vi "move_4b.vi"(6 "Array 5":i32[](array[numeric]), 7 "Array in":i32[](array[numeric]), 9 "Array 3":i32[](array[numeric]), 10 "Enum 4":T1(ring), 11 "Enum in":enum16{"move4", "move4_1", "move4_2"}(ring)) -> (1 "Array 4":i32[](array[numeric]), 2 "Enum 3":T2(ring), 3 "Enum out":enum16{"move4", "move4_1", "move4_2"}(ring), 4 "Array 6":i32[](array[numeric]), 5 "Array out":i32[](array[numeric]))   [LabVIEW 2016]
uses:
  <vilib>/NXT/Block Support/NXT_OutputPort.ctl
  <vilib>/NXT/NXTIO Xnodes/NXTIONodeSubVIs/NXTStopMotors.vi
  <vilib>/NXT/NXTIO Xnodes/NXTIONodeSubVIs/NXTMotorRunDistance.vi
  <vilib>/NXT/NXTIO Xnodes/NXTIONodeSubVIs/LEGOMotorStatus.vi
  <vilib>/NXT/NXTIO Xnodes/NXTIONodeSubVIs/NXTMoveMotors.vi
  <vilib>/NXT/NXTIO Xnodes/NXTIONodeSubVIs/LEGOResetMotors.vi
  <vilib>/NXT/Subs/LVHSConnector.ctl
  <vilib>/NXT/NXTIO Xnodes/AddressXNode/NXTIOAddress.xnode
  <vilib>/NXT/NXTIO Xnodes/NXTIOXNode/NXTIO.xnode
  <vilib>/NXT/LegoClasses/BrickReference/BrickReference.lvclass
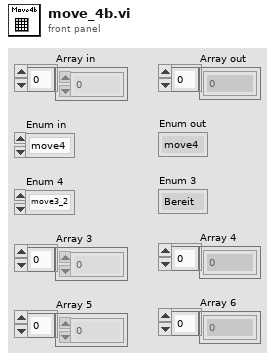
[diagram p1: front panel]
types:
  T1 = enum16{"move3_2", "move3_3", "move3_4", "move3_5"}
  T2 = enum16{"Bereit", "Move 1", "Reference_pos", "Wait", "row1_check", "row2_check", "row3_check", "return", "move2", "move3", "move4", "move5", "end"}
  T3 = enum16{"forward", "right", "mark", "pause", "up", "return", "end"}
  T4 = typedef "NXT_OutputPort.ctl" = u8
  T5 = cluster{"Output Port":T4, "Output Port 2":T4, "Output Port 3":T4}
  T6 = enum16{"forward", "mark", "pause", "up", "return", "end"}
  T7 = typedef "LVHSConnector.ctl" = refnum<class "BrickReference.lvclass">
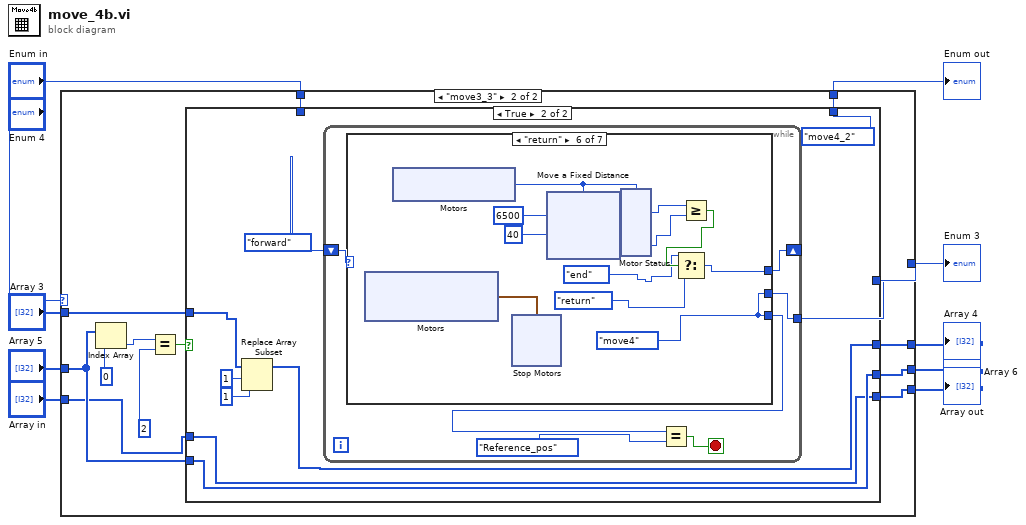
[diagram p0: block diagram]
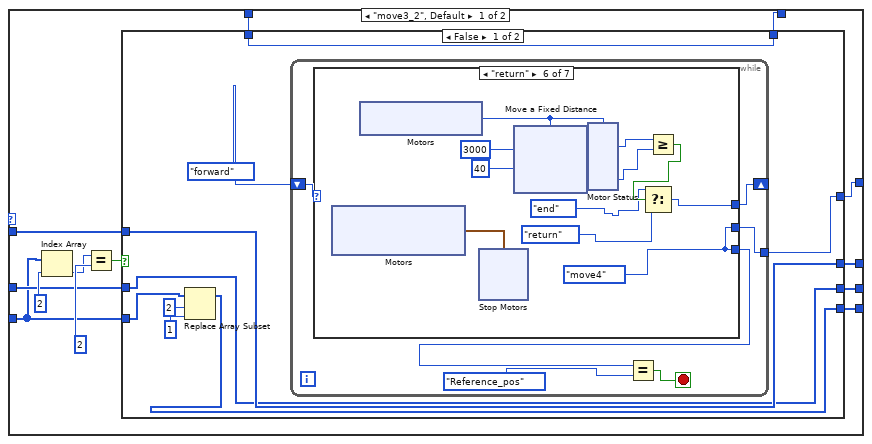
[diagram p2: hidden frame]
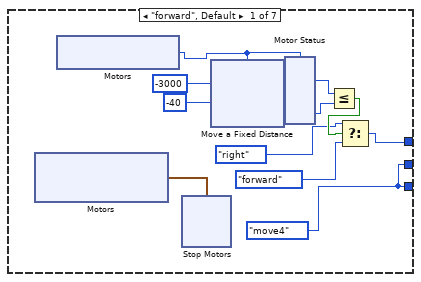
[diagram p3: hidden frame]
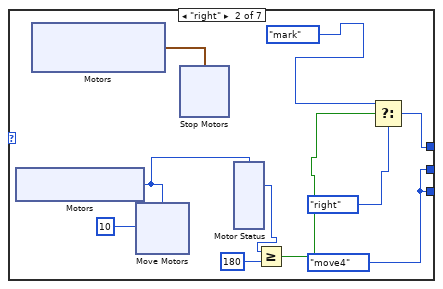
[diagram p4: hidden frame]
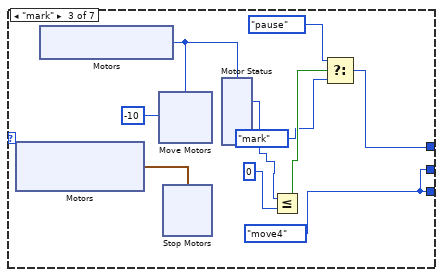
[diagram p5: hidden frame]
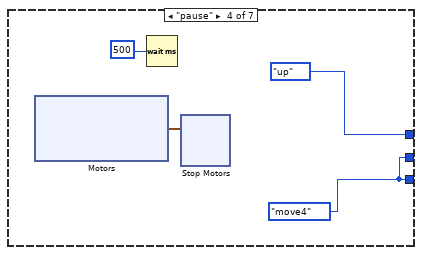
[diagram p6: hidden frame]
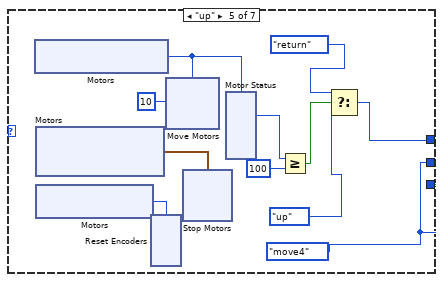
[diagram p7: hidden frame]
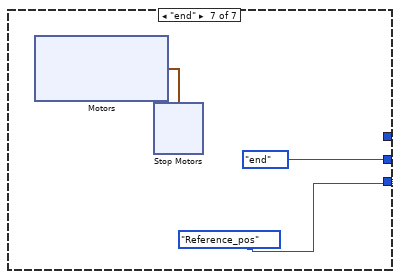
[diagram p8: hidden frame]
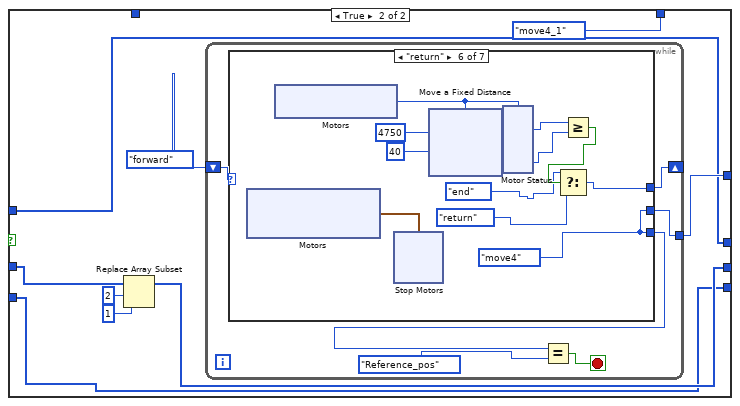
[diagram p9: hidden frame]
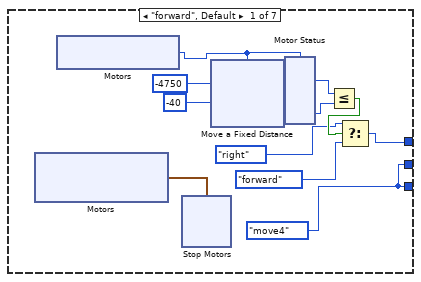
[diagram p10: hidden frame]
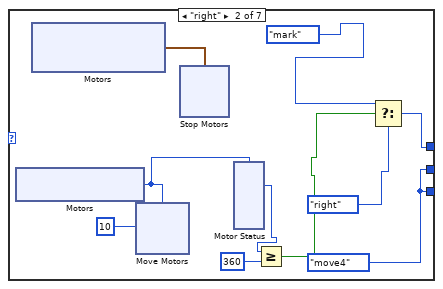
[diagram p11: hidden frame]
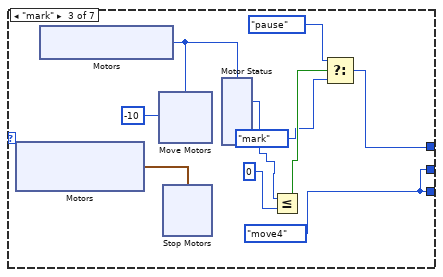
[diagram p12: hidden frame]
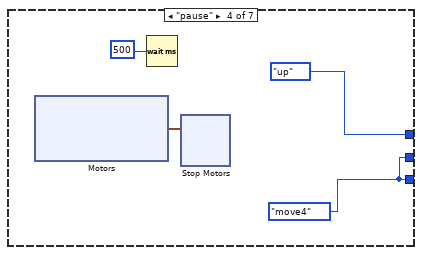
[diagram p13: hidden frame]
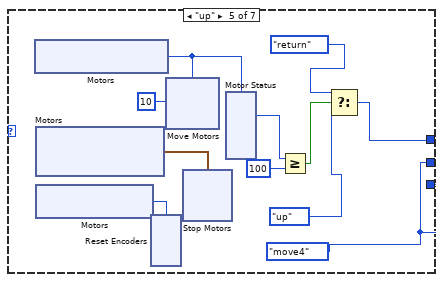
[diagram p14: hidden frame]
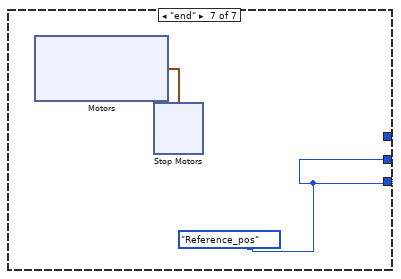
[diagram p15: hidden frame]
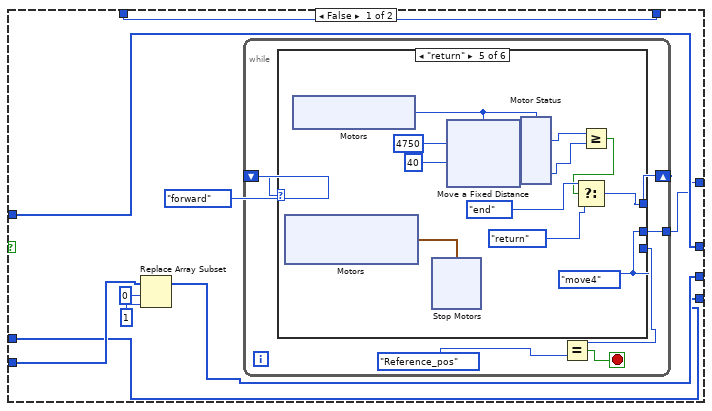
[diagram p16: hidden frame]
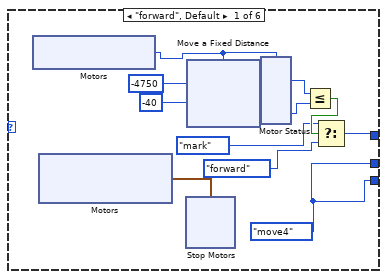
[diagram p17: hidden frame]
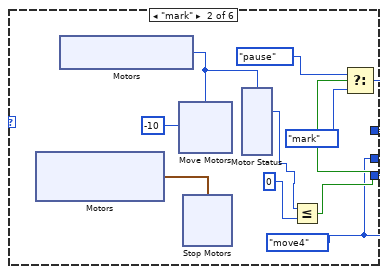
[diagram p18: hidden frame]
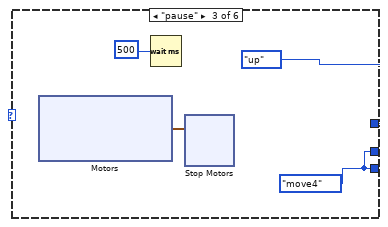
[diagram p19: hidden frame]
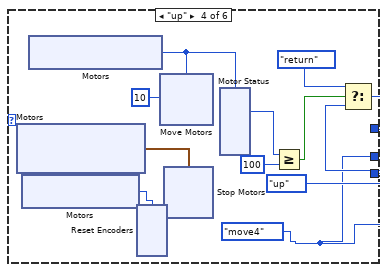
[diagram p20: hidden frame]
diagram:
  n1 = case shown="\"move3_3\"" "Enum 4" {
    tunnel: [w22 w450] -> w2
    tunnel: [w21 w449] -> w3
    tunnel: "Enum in" -> [w20 w448]
    tunnel: [w18 w442] -> w5
    tunnel: "Array 5" -> [w17 w441]
    tunnel: [w14 w443] -> w7
    tunnel: "Array 3" -> [w13 w444]
    tunnel: [w12 w440] -> w9
    tunnel: "Array in" -> [w11 w439]
    frame "move3_2", Default {
      n2 = Index Array(array=w11, index=2) -> (element=w16:i32)
      n3 = Equal?(x=w16, y=2 ("element")) -> (x = y?=w15:bool)
      n4 = case shown="False" w15 {
        tunnel: [w28 w239] -> w22
        tunnel: [w29 enum16{"move4", "move4_1", "move4_2"}."move4_1"] -> w21
        tunnel: w20 -> [w29 _]
        tunnel: [w24 w237] -> w18
        tunnel: w17 -> [w24 w238]
        tunnel: [w27 w233] -> w14
        tunnel: w13 -> [w27 w233]
        tunnel: [w25 w234] -> w12
        tunnel: w11 -> [w26 w234]
        frame False {
          n5 = Replace Array Subset(array=w26, new element=1 ("new element/subarray"), index=2) -> (w25:i32[])
          n6 = while {
            shift-right: [w34] -> _
            shift-left: T3."forward" -> [w35]
            tunnel: [w33] -> w28
            stop <- w37 stop-if-true
            n7 = case shown="\"return\"" w35 {
              tunnel: [w39 w76 w108 T3."up" w151 w187 _] -> w34
              tunnel: [w48 w75 w107 w139 w150 w196 T2."Reference_pos"] -> w38
              tunnel: [w48 w75 w107 w139 w150 w196 T2."end"] -> w33
              frame "forward", Default {
                w44 = -3000 ("Distance 1")
                w48 = T2."move4"
                n8 = xnode "Motors"() -> ("Motor"=w49:cluster{"Port":T4, "Port":T4})
                n9 = xnode "Motors"() -> ("Motor"=w43:T4)
                n10 = xnode "Stop Motors"("Motors"=w49) -> ()  [unwired: 1 in, 1 out]
                n11 = xnode "Move a Fixed Distance"("Speed 1"=i8 -40, "Distance 1"=w44, "Motors"=w43) -> ("NXT/EV3"=w45:T7)  [unwired: 1 in]
                n12 = xnode "Motor Status"("Motors"=w43, "NXT/EV3"=w45) -> ("Position 1"=w46:i32)  [unwired: 2 out]
                n13 = Less Or Equal?(x=w46, y=w44) -> (x <= y?=w42:bool)
                n14 = Select(t=T3."right", s=w42, f=T3."forward") -> (s? t:f=w39:T3)
              }
              frame "right" {
                w75 = T2."move4"
                n15 = xnode "Motors"() -> ("Motor"=w84:T4)
                n16 = xnode "Motors"() -> ("Motor"=w83:cluster{"Port":T4, "Port":T4})
                n17 = xnode "Move Motors"("Power/Speed 1"=i8 10, "Motors"=w84) -> ()  [unwired: 1 in, 1 out]
                n18 = xnode "Stop Motors"("Motors"=w83) -> ()  [unwired: 1 in, 1 out]
                n19 = xnode "Motor Status"("Motors"=w84) -> ("Position 1"=w81:i32)  [unwired: 1 in, 2 out]
                n20 = Greater Or Equal?(x=w81, y=180) -> (x >= y?=w80:bool)
                n21 = Select(t=T3."mark", s=w80, f=T3."right") -> (s? t:f=w76:T3)
              }
              frame "mark" {
                w107 = T2."move4"
                n22 = xnode "Motors"() -> ("Motor"=w116:cluster{"Port":T4, "Port":T4})
                n23 = xnode "Motors"() -> ("Motor"=w114:T4)
                n24 = xnode "Move Motors"("Power/Speed 1"=i8 -10, "Motors"=w114) -> ()  [unwired: 1 in, 1 out]
                n25 = xnode "Stop Motors"("Motors"=w116) -> ()  [unwired: 1 in, 1 out]
                n26 = xnode "Motor Status"("Motors"=w114) -> ("Position 1"=w113:i32)  [unwired: 1 in, 2 out]
                n27 = Less Or Equal?(x=w113, y=0) -> (x <= y?=w111:bool)
                n28 = Select(t=T3."pause", s=w111, f=T3."mark") -> (s? t:f=w108:T3)
              }
              frame "pause" {
                w139 = T2."move4"
                n29 = xnode "Motors"() -> ("Motor"=w142:cluster{"Port":T4, "Port":T4, "Port":T4})
                n30 = Wait (ms)(milliseconds to wait=u32 500 ("millisecond timer value")) -> ()  [unwired: 1 out]
                n31 = xnode "Stop Motors"("Motors"=w142) -> ()  [unwired: 1 in, 1 out]
              }
              frame "up" {
                w150 = T2."move4"
                n32 = xnode "Motors"() -> ("Motor"=w155:T4)
                n33 = xnode "Motors"() -> ("Motor"=w158:cluster{"Port":T4, "Port":T4})
                n34 = xnode "Motors"() -> ("Motor"=w149:T4)
                n35 = xnode "Reset Encoders"("Motors"=w149) -> ()  [unwired: 1 in, 1 out]
                n36 = xnode "Move Motors"("Power/Speed 1"=i8 10, "Motors"=w155) -> ()  [unwired: 1 in, 1 out]
                n37 = xnode "Stop Motors"("Motors"=w158) -> ()  [unwired: 1 in, 1 out]
                n38 = xnode "Motor Status"("Motors"=w155) -> ("Position 1"=w156:i32)  [unwired: 1 in, 2 out]
                n39 = Greater Or Equal?(x=w156, y=100) -> (x >= y?=w157:bool)
                n40 = Select(t=T3."return", s=w157, f=T3."up") -> (s? t:f=w151:T3)
              }
              frame "return" {
                w191 = 3000 ("Distance 1")
                w196 = T2."move4"
                n41 = xnode "Motors"() -> ("Motor"=w197:cluster{"Port":T4, "Port":T4})
                n42 = xnode "Motors"() -> ("Motor"=w194:T4)
                n43 = xnode "Stop Motors"("Motors"=w197) -> ()  [unwired: 1 in, 1 out]
                n44 = xnode "Move a Fixed Distance"("Speed 1"=i8 40, "Distance 1"=w191, "Motors"=w194) -> ("NXT/EV3"=w193:T7)  [unwired: 1 in]
                n45 = xnode "Motor Status"("Motors"=w194, "NXT/EV3"=w193) -> ("Position 1"=w192:i32)  [unwired: 2 out]
                n46 = Greater Or Equal?(x=w192, y=w191) -> (x >= y?=w190:bool)
                n47 = Select(t=T3."end", s=w190, f=T3."return") -> (s? t:f=w187:T3)
              }
              frame "end" {
                n48 = xnode "Motors"() -> ("Motor"=w224:cluster{"Port":T4, "Port":T4, "Port":T4})
                n49 = xnode "Stop Motors"("Motors"=w224) -> ()  [unwired: 1 in, 1 out]
              }
            }
            n50 = Equal?(x=w38, y=T2."Reference_pos") -> (x = y?=w37:bool)
          }
        }
        frame True {
          n51 = Replace Array Subset(array=w238, new element=1 ("new element/subarray"), index=2) -> (w237:i32[])
          n52 = while {
            shift-right: [w242] -> _
            shift-left: T3."forward" -> [w243]
            tunnel: [w241] -> w239
            stop <- w245 stop-if-true
            n53 = case shown="\"return\"" w243 {
              tunnel: [w247 w284 w316 T3."up" w359 w395 _] -> w242
              tunnel: [w256 w283 w315 w347 w358 w404 w431] -> w246
              tunnel: [w256 w283 w315 w347 w358 w404 w431] -> w241
              frame "forward", Default {
                w252 = -4750 ("Distance 1")
                w256 = T2."move4"
                n54 = xnode "Motors"() -> ("Motor"=w257:cluster{"Port":T4, "Port":T4})
                n55 = xnode "Motors"() -> ("Motor"=w251:T4)
                n56 = xnode "Stop Motors"("Motors"=w257) -> ()  [unwired: 1 in, 1 out]
                n57 = xnode "Move a Fixed Distance"("Speed 1"=i8 -40, "Distance 1"=w252, "Motors"=w251) -> ("NXT/EV3"=w253:T7)  [unwired: 1 in]
                n58 = xnode "Motor Status"("Motors"=w251, "NXT/EV3"=w253) -> ("Position 1"=w254:i32)  [unwired: 2 out]
                n59 = Less Or Equal?(x=w254, y=w252) -> (x <= y?=w250:bool)
                n60 = Select(t=T3."right", s=w250, f=T3."forward") -> (s? t:f=w247:T3)
              }
              frame "right" {
                w283 = T2."move4"
                n61 = xnode "Motors"() -> ("Motor"=w292:T4)
                n62 = xnode "Motors"() -> ("Motor"=w291:cluster{"Port":T4, "Port":T4})
                n63 = xnode "Move Motors"("Power/Speed 1"=i8 10, "Motors"=w292) -> ()  [unwired: 1 in, 1 out]
                n64 = xnode "Stop Motors"("Motors"=w291) -> ()  [unwired: 1 in, 1 out]
                n65 = xnode "Motor Status"("Motors"=w292) -> ("Position 1"=w289:i32)  [unwired: 1 in, 2 out]
                n66 = Greater Or Equal?(x=w289, y=360) -> (x >= y?=w288:bool)
                n67 = Select(t=T3."mark", s=w288, f=T3."right") -> (s? t:f=w284:T3)
              }
              frame "mark" {
                w315 = T2."move4"
                n68 = xnode "Motors"() -> ("Motor"=w324:cluster{"Port":T4, "Port":T4})
                n69 = xnode "Motors"() -> ("Motor"=w322:T4)
                n70 = xnode "Move Motors"("Power/Speed 1"=i8 -10, "Motors"=w322) -> ()  [unwired: 1 in, 1 out]
                n71 = xnode "Stop Motors"("Motors"=w324) -> ()  [unwired: 1 in, 1 out]
                n72 = xnode "Motor Status"("Motors"=w322) -> ("Position 1"=w321:i32)  [unwired: 1 in, 2 out]
                n73 = Less Or Equal?(x=w321, y=0) -> (x <= y?=w319:bool)
                n74 = Select(t=T3."pause", s=w319, f=T3."mark") -> (s? t:f=w316:T3)
              }
              frame "pause" {
                w347 = T2."move4"
                n75 = xnode "Motors"() -> ("Motor"=w350:cluster{"Port":T4, "Port":T4, "Port":T4})
                n76 = Wait (ms)(milliseconds to wait=u32 500 ("millisecond timer value")) -> ()  [unwired: 1 out]
                n77 = xnode "Stop Motors"("Motors"=w350) -> ()  [unwired: 1 in, 1 out]
              }
              frame "up" {
                w358 = T2."move4"
                n78 = xnode "Motors"() -> ("Motor"=w363:T4)
                n79 = xnode "Motors"() -> ("Motor"=w366:cluster{"Port":T4, "Port":T4})
                n80 = xnode "Motors"() -> ("Motor"=w357:T4)
                n81 = xnode "Reset Encoders"("Motors"=w357) -> ()  [unwired: 1 in, 1 out]
                n82 = xnode "Move Motors"("Power/Speed 1"=i8 10, "Motors"=w363) -> ()  [unwired: 1 in, 1 out]
                n83 = xnode "Stop Motors"("Motors"=w366) -> ()  [unwired: 1 in, 1 out]
                n84 = xnode "Motor Status"("Motors"=w363) -> ("Position 1"=w364:i32)  [unwired: 1 in, 2 out]
                n85 = Greater Or Equal?(x=w364, y=100) -> (x >= y?=w365:bool)
                n86 = Select(t=T3."return", s=w365, f=T3."up") -> (s? t:f=w359:T3)
              }
              frame "return" {
                w399 = 4750 ("Distance 1")
                w404 = T2."move4"
                n87 = xnode "Motors"() -> ("Motor"=w405:cluster{"Port":T4, "Port":T4})
                n88 = xnode "Motors"() -> ("Motor"=w402:T4)
                n89 = xnode "Stop Motors"("Motors"=w405) -> ()  [unwired: 1 in, 1 out]
                n90 = xnode "Move a Fixed Distance"("Speed 1"=i8 40, "Distance 1"=w399, "Motors"=w402) -> ("NXT/EV3"=w401:T7)  [unwired: 1 in]
                n91 = xnode "Motor Status"("Motors"=w402, "NXT/EV3"=w401) -> ("Position 1"=w400:i32)  [unwired: 2 out]
                n92 = Greater Or Equal?(x=w400, y=w399) -> (x >= y?=w398:bool)
                n93 = Select(t=T3."end", s=w398, f=T3."return") -> (s? t:f=w395:T3)
              }
              frame "end" {
                w431 = T2."Reference_pos"
                n94 = xnode "Motors"() -> ("Motor"=w432:cluster{"Port":T4, "Port":T4, "Port":T4})
                n95 = xnode "Stop Motors"("Motors"=w432) -> ()  [unwired: 1 in, 1 out]
              }
            }
            n96 = Equal?(x=w246, y=T2."Reference_pos") -> (x = y?=w245:bool)
          }
        }
      }
    }
    frame "move3_3" {
      n97 = Index Array(array=w441, index=0) -> (element=w446:i32)
      n98 = Equal?(x=w446, y=2 ("element")) -> (x = y?=w445:bool)
      n99 = case shown="True" w445 {
        tunnel: [w452 w634] -> w450
        tunnel: [w460 enum16{"move4", "move4_1", "move4_2"}."move4_2"] -> w449
        tunnel: w448 -> [w460 _]
        tunnel: w444 -> [w453 w632]
        tunnel: [w453 w630] -> w443
        tunnel: [w455 w629] -> w442
        tunnel: w441 -> [w456 w629]
        tunnel: [w454 w628] -> w440
        tunnel: w439 -> [w454 w628]
        frame False {
          n100 = Replace Array Subset(array=w456, new element=1 ("new element/subarray"), index=0) -> (w455:i32[])
          n101 = while {
            shift-right: [w466] -> _
            shift-left: T6."forward" -> [w465]
            tunnel: [w461] -> w452
            stop <- w463 stop-if-true
            n102 = case shown="\"return\"" w465 {
              tunnel: [w467 w510 T6."up" w552 w584 _] -> w466
              tunnel: [w476 w503 w535 w546 w592 T2."Reference_pos"] -> w464
              tunnel: [w476 w503 w535 w546 w592 T2."end"] -> w461
              frame "forward", Default {
                w472 = -4750 ("Distance 1")
                w476 = T2."move4"
                n103 = xnode "Motors"() -> ("Motor"=w471:T4)
                n104 = xnode "Motors"() -> ("Motor"=w477:cluster{"Port":T4, "Port":T4})
                n105 = xnode "Stop Motors"("Motors"=w477) -> ()  [unwired: 1 in, 1 out]
                n106 = xnode "Move a Fixed Distance"("Speed 1"=i8 -40, "Distance 1"=w472, "Motors"=w471) -> ("NXT/EV3"=w473:T7)  [unwired: 1 in]
                n107 = xnode "Motor Status"("Motors"=w471, "NXT/EV3"=w473) -> ("Position 1"=w474:i32)  [unwired: 2 out]
                n108 = Less Or Equal?(x=w474, y=w472) -> (x <= y?=w470:bool)
                n109 = Select(t=T6."mark", s=w470, f=T6."forward") -> (s? t:f=w467:T6)
              }
              frame "mark" {
                w503 = T2."move4"
                n110 = xnode "Motors"() -> ("Motor"=w512:cluster{"Port":T4, "Port":T4})
                n111 = xnode "Motors"() -> ("Motor"=w507:T4)
                n112 = xnode "Move Motors"("Power/Speed 1"=i8 -10, "Motors"=w507) -> ()  [unwired: 1 in, 1 out]
                n113 = xnode "Stop Motors"("Motors"=w512) -> ()  [unwired: 1 in, 1 out]
                n114 = xnode "Motor Status"("Motors"=w507) -> ("Position 1"=w506:i32)  [unwired: 1 in, 2 out]
                n115 = Less Or Equal?(x=w506, y=0) -> (x <= y?=w504:bool)
                n116 = Select(t=T6."pause", s=w504, f=T6."mark") -> (s? t:f=w510:T6)
              }
              frame "pause" {
                w535 = T2."move4"
                n117 = xnode "Motors"() -> ("Motor"=w538:cluster{"Port":T4, "Port":T4, "Port":T4})
                n118 = Wait (ms)(milliseconds to wait=u32 500 ("millisecond timer value")) -> ()  [unwired: 1 out]
                n119 = xnode "Stop Motors"("Motors"=w538) -> ()  [unwired: 1 in, 1 out]
              }
              frame "up" {
                w546 = T2."move4"
                n120 = xnode "Motors"() -> ("Motor"=w554:cluster{"Port":T4, "Port":T4})
                n121 = xnode "Motors"() -> ("Motor"=w545:T4)
                n122 = xnode "Motors"() -> ("Motor"=w548:T4)
                n123 = xnode "Reset Encoders"("Motors"=w545) -> ()  [unwired: 1 in, 1 out]
                n124 = xnode "Move Motors"("Power/Speed 1"=i8 10, "Motors"=w548) -> ()  [unwired: 1 in, 1 out]
                n125 = xnode "Stop Motors"("Motors"=w554) -> ()  [unwired: 1 in, 1 out]
                n126 = xnode "Motor Status"("Motors"=w548) -> ("Position 1"=w549:i32)  [unwired: 1 in, 2 out]
                n127 = Greater Or Equal?(x=w549, y=100) -> (x >= y?=w553:bool)
                n128 = Select(t=T6."return", s=w553, f=T6."up") -> (s? t:f=w552:T6)
              }
              frame "return" {
                w587 = 4750 ("Distance 1")
                w592 = T2."move4"
                n129 = xnode "Motors"() -> ("Motor"=w593:cluster{"Port":T4, "Port":T4})
                n130 = xnode "Motors"() -> ("Motor"=w590:T4)
                n131 = xnode "Stop Motors"("Motors"=w593) -> ()  [unwired: 1 in, 1 out]
                n132 = xnode "Move a Fixed Distance"("Speed 1"=i8 40, "Distance 1"=w587, "Motors"=w590) -> ("NXT/EV3"=w589:T7)  [unwired: 1 in]
                n133 = xnode "Motor Status"("Motors"=w590, "NXT/EV3"=w589) -> ("Position 1"=w588:i32)  [unwired: 2 out]
                n134 = Greater Or Equal?(x=w588, y=w587) -> (x >= y?=w583:bool)
                n135 = Select(t=T6."end", s=w583, f=T6."return") -> (s? t:f=w584:T6)
              }
              frame "end" {
                n136 = xnode "Motors"() -> ("Motor"=w621:cluster{"Port":T4, "Port":T4, "Port":T4})
                n137 = xnode "Stop Motors"("Motors"=w621) -> ()  [unwired: 1 in, 1 out]
              }
            }
            n138 = Equal?(x=w464, y=T2."Reference_pos") -> (x = y?=w463:bool)
          }
        }
        frame True {
          n139 = Replace Array Subset(array=w632, new element=1 ("new element/subarray"), index=1) -> (w630:i32[])
          n140 = while {
            shift-right: [w638] -> _
            shift-left: T3."forward" -> [w639]
            tunnel: [w637] -> w634
            stop <- w641 stop-if-true
            n141 = case shown="\"return\"" w639 {
              tunnel: [w643 w680 w712 T3."up" w755 w791 _] -> w638
              tunnel: [w652 w679 w711 w743 w754 w800 w827] -> w642
              tunnel: [w652 w679 w711 w743 w754 w800 w827] -> w637
              frame "forward", Default {
                w648 = -6500 ("Distance 1")
                w652 = T2."move4"
                n142 = xnode "Motors"() -> ("Motor"=w653:cluster{"Port":T4, "Port":T4})
                n143 = xnode "Motors"() -> ("Motor"=w647:T4)
                n144 = xnode "Stop Motors"("Motors"=w653) -> ()  [unwired: 1 in, 1 out]
                n145 = xnode "Move a Fixed Distance"("Speed 1"=i8 -40, "Distance 1"=w648, "Motors"=w647) -> ("NXT/EV3"=w649:T7)  [unwired: 1 in]
                n146 = xnode "Motor Status"("Motors"=w647, "NXT/EV3"=w649) -> ("Position 1"=w650:i32)  [unwired: 2 out]
                n147 = Less Or Equal?(x=w650, y=w648) -> (x <= y?=w646:bool)
                n148 = Select(t=T3."right", s=w646, f=T3."forward") -> (s? t:f=w643:T3)
              }
              frame "right" {
                w679 = T2."move4"
                n149 = xnode "Motors"() -> ("Motor"=w688:T4)
                n150 = xnode "Motors"() -> ("Motor"=w687:cluster{"Port":T4, "Port":T4})
                n151 = xnode "Move Motors"("Power/Speed 1"=i8 10, "Motors"=w688) -> ()  [unwired: 1 in, 1 out]
                n152 = xnode "Stop Motors"("Motors"=w687) -> ()  [unwired: 1 in, 1 out]
                n153 = xnode "Motor Status"("Motors"=w688) -> ("Position 1"=w685:i32)  [unwired: 1 in, 2 out]
                n154 = Greater Or Equal?(x=w685, y=180) -> (x >= y?=w684:bool)
                n155 = Select(t=T3."mark", s=w684, f=T3."right") -> (s? t:f=w680:T3)
              }
              frame "mark" {
                w711 = T2."move4"
                n156 = xnode "Motors"() -> ("Motor"=w720:cluster{"Port":T4, "Port":T4})
                n157 = xnode "Motors"() -> ("Motor"=w718:T4)
                n158 = xnode "Move Motors"("Power/Speed 1"=i8 -10, "Motors"=w718) -> ()  [unwired: 1 in, 1 out]
                n159 = xnode "Stop Motors"("Motors"=w720) -> ()  [unwired: 1 in, 1 out]
                n160 = xnode "Motor Status"("Motors"=w718) -> ("Position 1"=w717:i32)  [unwired: 1 in, 2 out]
                n161 = Less Or Equal?(x=w717, y=0) -> (x <= y?=w715:bool)
                n162 = Select(t=T3."pause", s=w715, f=T3."mark") -> (s? t:f=w712:T3)
              }
              frame "pause" {
                w743 = T2."move4"
                n163 = xnode "Motors"() -> ("Motor"=w746:cluster{"Port":T4, "Port":T4, "Port":T4})
                n164 = Wait (ms)(milliseconds to wait=u32 500 ("millisecond timer value")) -> ()  [unwired: 1 out]
                n165 = xnode "Stop Motors"("Motors"=w746) -> ()  [unwired: 1 in, 1 out]
              }
              frame "up" {
                w754 = T2."move4"
                n166 = xnode "Motors"() -> ("Motor"=w759:T4)
                n167 = xnode "Motors"() -> ("Motor"=w762:cluster{"Port":T4, "Port":T4})
                n168 = xnode "Motors"() -> ("Motor"=w753:T4)
                n169 = xnode "Reset Encoders"("Motors"=w753) -> ()  [unwired: 1 in, 1 out]
                n170 = xnode "Move Motors"("Power/Speed 1"=i8 10, "Motors"=w759) -> ()  [unwired: 1 in, 1 out]
                n171 = xnode "Stop Motors"("Motors"=w762) -> ()  [unwired: 1 in, 1 out]
                n172 = xnode "Motor Status"("Motors"=w759) -> ("Position 1"=w760:i32)  [unwired: 1 in, 2 out]
                n173 = Greater Or Equal?(x=w760, y=100) -> (x >= y?=w761:bool)
                n174 = Select(t=T3."return", s=w761, f=T3."up") -> (s? t:f=w755:T3)
              }
              frame "return" {
                w795 = 6500 ("Distance 1")
                w800 = T2."move4"
                n175 = xnode "Motors"() -> ("Motor"=w801:cluster{"Port":T4, "Port":T4})
                n176 = xnode "Motors"() -> ("Motor"=w798:T4)
                n177 = xnode "Stop Motors"("Motors"=w801) -> ()  [unwired: 1 in, 1 out]
                n178 = xnode "Move a Fixed Distance"("Speed 1"=i8 40, "Distance 1"=w795, "Motors"=w798) -> ("NXT/EV3"=w797:T7)  [unwired: 1 in]
                n179 = xnode "Motor Status"("Motors"=w798, "NXT/EV3"=w797) -> ("Position 1"=w796:i32)  [unwired: 2 out]
                n180 = Greater Or Equal?(x=w796, y=w795) -> (x >= y?=w794:bool)
                n181 = Select(t=T3."end", s=w794, f=T3."return") -> (s? t:f=w791:T3)
              }
              frame "end" {
                w827 = T2."Reference_pos"
                n182 = xnode "Motors"() -> ("Motor"=w828:cluster{"Port":T4, "Port":T4, "Port":T4})
                n183 = xnode "Stop Motors"("Motors"=w828) -> ()  [unwired: 1 in, 1 out]
              }
            }
            n184 = Equal?(x=w642, y=T2."Reference_pos") -> (x = y?=w641:bool)
          }
        }
      }
    }
  }
  "Array out" <- w9
  "Array 4" <- w7
  "Array 6" <- w5
  "Enum out" <- w3
  "Enum 3" <- w2
